vi "_Get VIs in Project.vi"(8 "error in (no error)":errorcluster, 11 "project":refnum<vi>) -> (0 "error out":errorcluster, 2 "Array of VIs":T1[](array[typedef]), 3 "project out":refnum<vi>)   [LabVIEW 2017, in "CSM_ExampleBrowser.lvlib"]
uses:
  CSM_ExampleBrowser.lvlib
  controls/BMark_VI_Identifier.ctl
  <vilib>/addons/analyzer/_analyzerctrls.llb/VIAnCtl Analysis App Info.ctl
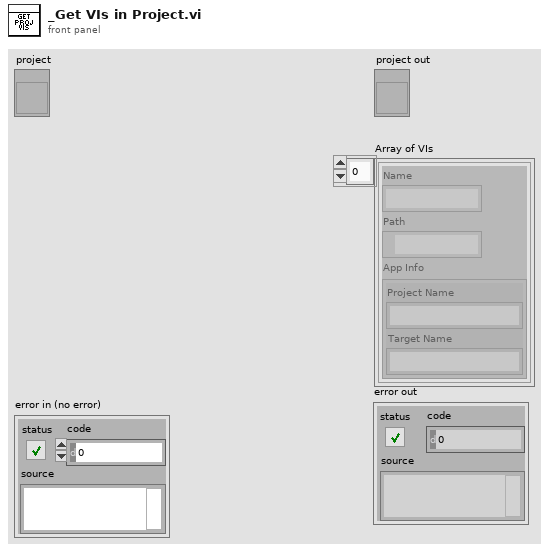
[diagram p1: front panel]
types:
  T1 = typedef "CSM_ExampleBrowser.lvlib/BMark_VI_Identifier.ctl" = cluster{"Name":string, "Path":path, "App Info":T2}
  T2 = typedef "VIAnCtl Analysis App Info.ctl" = cluster{"Project Name":string, "Target Name":string}
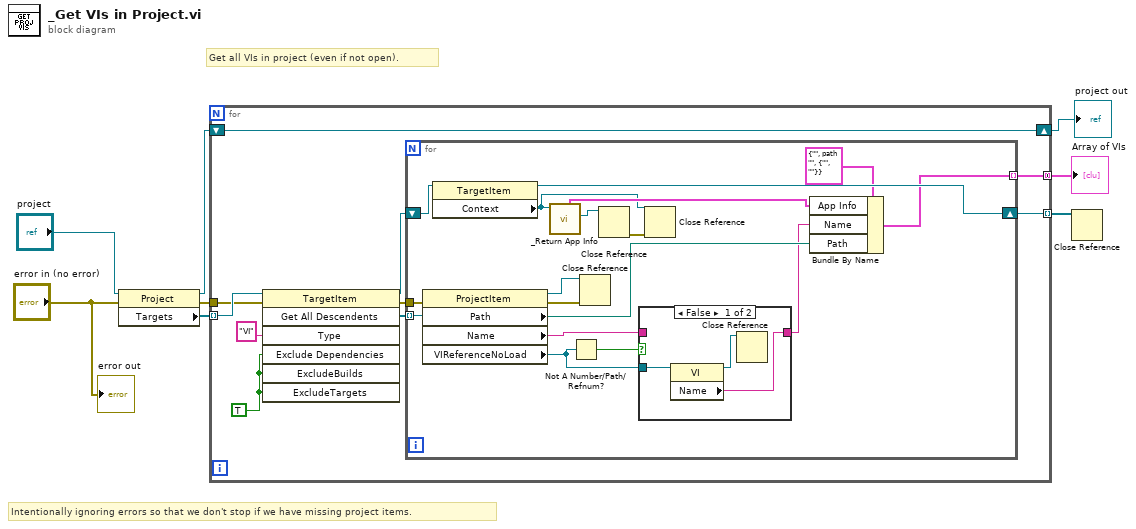
[diagram p0: block diagram]
diagram:
  # "Intentionally ignoring errors so that we don't stop if we have missing project items."
  # "Get all VIs in project (even if not open)."
  n1 = property class="Project"(reference="project", error in="error in (no error)") -> (reference out=w2:refnum<vi>, error out=w6:errorcluster, "Targets"=w8:refnum<vi>[])
  n2 = for {
    tunnel: w8 -> [w18] mode=indexing
    tunnel: [w12] -> w5 mode=indexing
    tunnel: [w11] -> w4 mode=concatenating
    tunnel: w6 -> [w15]
    shift-right: [w9] -> w1
    shift-left: w2 -> [w9]
    w10 = TRUE ("ExcludeDependencies")
    n3 = invoke class="TargetItem" method="Get All Descendents"(reference=w18, error in=w15, "Type"="VI", "Exclude Dependencies"=w10, "ExcludeBuilds"=w10, "ExcludeTargets"=w10) -> (reference out=w13:refnum<vi>, error out=w14:errorcluster, "All Descendents"=w16:refnum<vi>[])  [unwired: 1 in, 4 out]
    n4 = for {
      tunnel: w16 -> [w35] mode=indexing
      shift-right: [w30] -> w12
      shift-left: w13 -> [w31]
      tunnel: [w27] -> w11 mode=indexing
      tunnel: w14 -> [w34]
      n5 = property class="ProjectItem"(reference=w35, error in=w34) -> (reference out=w32:refnum<vi>, error out=w33:errorcluster, "Path"=w28:path, "Name"=w25:string, "VIReferenceNoLoad"=w24:refnum<vi>)
      n6 = property class="TargetItem"(reference=w31) -> (reference out=w30:refnum<vi>, "Context"=w19:refnum<vi>)  [unwired: 1 in, 1 out]
      n7 = call "_Return App Info.vi"("App Refnum in"=w19) -> ("App Refnum for Opening VI"=w21:refnum<vi>, "App Info"=w22:T2)  [unwired: 8 in, 1 out]
      n8 = Not A Number/Path/Refnum?(number/path/refnum=w24) -> (NaN/Path/Refnum?=w26:bool)
      n9 = Close Reference(reference=w32, error in (no error)=w33) -> ()  [unwired: 1 out]
      n10 = Close Reference(reference=w21) -> (error out=w20:errorcluster)  [unwired: 1 in]
      n11 = case shown="False" w26 {
        tunnel: w25 -> [_ w39]
        tunnel: [w37 w39] -> w23
        tunnel: w24 -> [w38 _]
        frame False {
          n12 = property class="VI"(reference=w38) -> (reference out=w36:refnum<vi>, "Name"=w37:string)  [unwired: 1 in, 1 out]
          n13 = Close Reference(reference=w36) -> ()  [unwired: 1 in, 1 out]
        }
        frame True {
        }
      }
      n14 = Close Reference(reference=w19, error in (no error)=w20) -> ()  [unwired: 1 out]
      n15 = Bundle By Name(cluster=T1 {"Name"="", "Path"=path "", "App Info"={"Project Name"="", "Target Name"=""}}, "App Info"=w22, "Name"=w23, "Path"=w28) -> (w27:T1)
    }
  }
  "Array of VIs" <- w4
  "project out" <- w1
  n16 = Close Reference(reference=w5) -> ()  [unwired: 1 in, 1 out]
  "error out" <- "error in (no error)"
